vi "Test_ItemInventory.vi"() -> ()   [LabVIEW 2016]
uses:
  Device Info.ctl
  Array Device Info.ctl
panel:
  out "array of devices":T1
  in  "Stop Button":bool
  out "error out":errorcluster
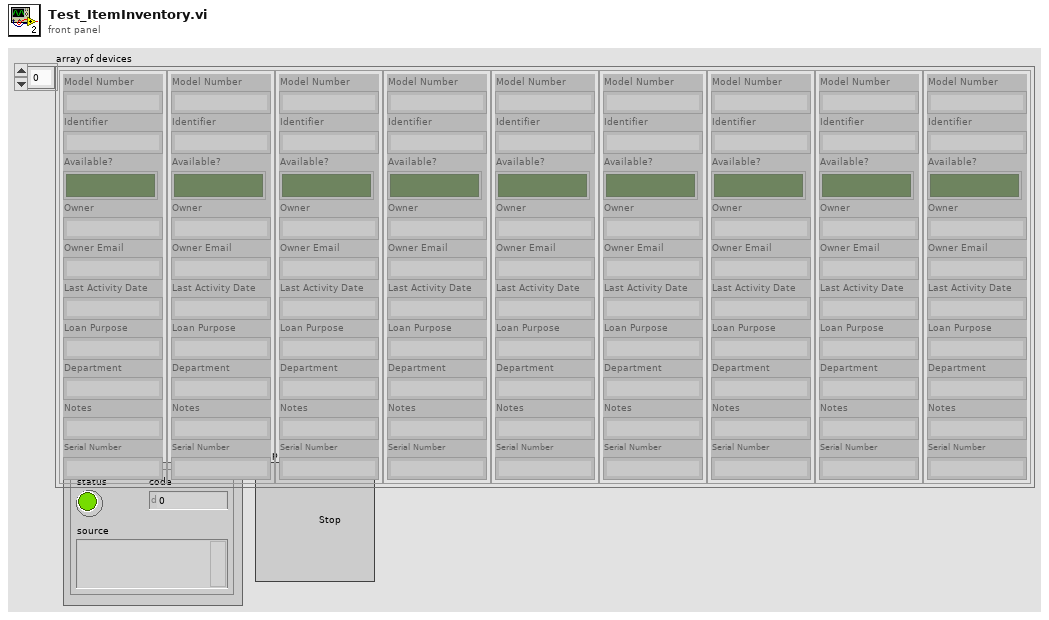
[diagram p1: front panel]
types:
  T1 = typedef "Array Device Info.ctl" = T2[]
  T2 = typedef "Device Info.ctl" = cluster{"Model Number":string, "Identifier":string, "Available?":bool, "Owner":string, "Owner Email":string, "Last Activity Date":string, "Loan Purpose":string, "Department":string, "Notes":string, "Serial Number":string}
  T3 = enum16{"Load Items", "Check Status", "Return Items", "Check Out Items", "Add New Item", "Get All Items", "Remove Item"}
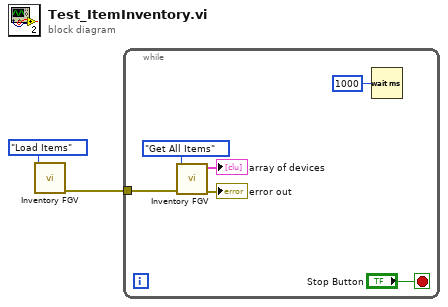
[diagram p0: block diagram]
diagram:
  n1 = call "Inventory FGV.vi"("Command"=T3."Load Items") -> ("error out"=w1:errorcluster)  [unwired: 7 in, 2 out]
  n2 = while {
    tunnel: w1 -> [w8]
    stop <- "Stop Button" stop-if-true
    n3 = call "Inventory FGV.vi"("error in"=w8, "Command"=T3."Get All Items") -> ("error out"=→"error out":errorcluster, "array of devices"=→"array of devices":T1)  [unwired: 6 in, 1 out]
    n4 = Wait (ms)(milliseconds to wait=u32 1000) -> ()  [unwired: 1 out]
  }
